vi "Measure.vi"(8 "Error In":errorcluster, 11 "Keithley 6482 In":refnum<visa-resource-name>) -> (0 "Error Out":errorcluster, 2 "Values":dbl[](array[numeric]), 3 "Keithley 6482 Out":refnum<visa-resource-name>)   [LabVIEW 2014, in "Keithley-6482-Visa.lvlib"]
uses:
  Keithley-6482-Visa.lvlib
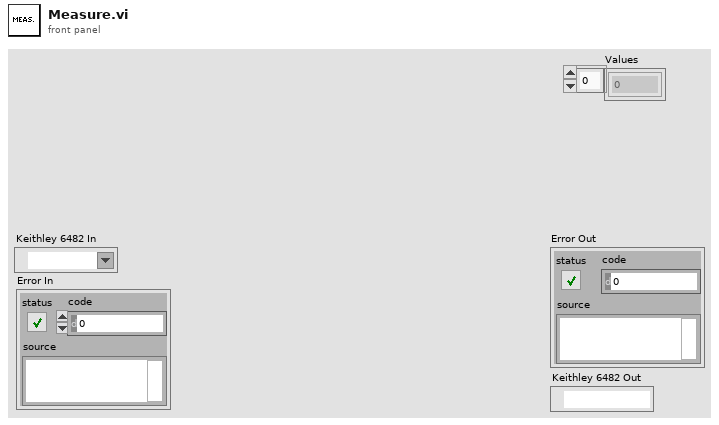
[diagram p1: front panel]
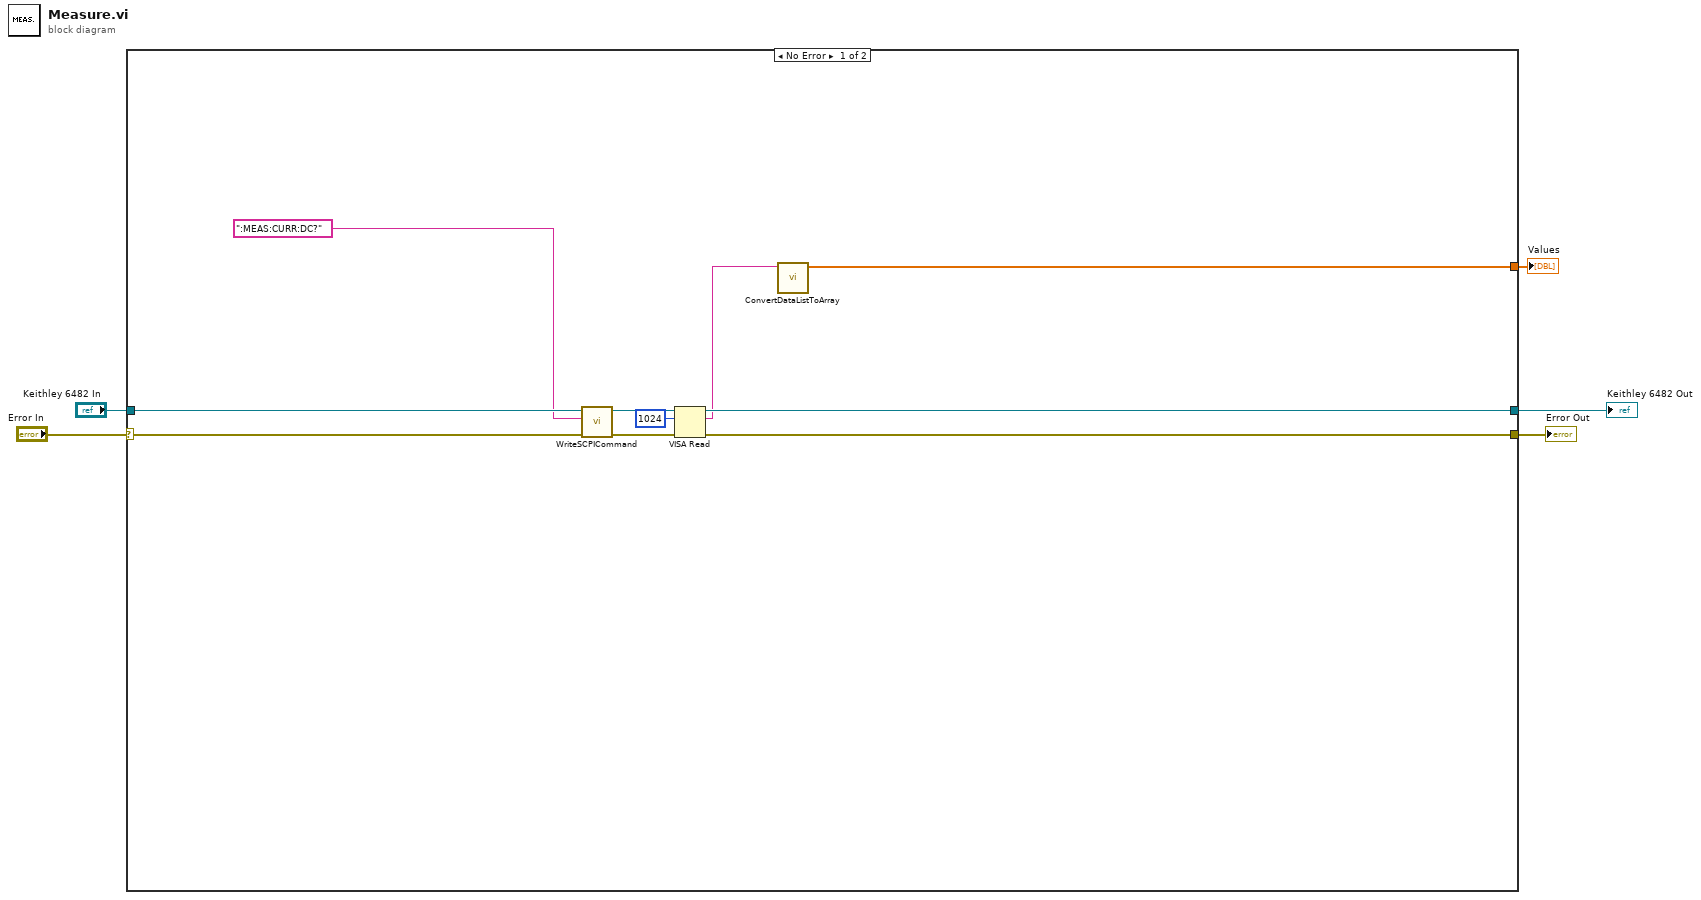
[diagram p0: block diagram]
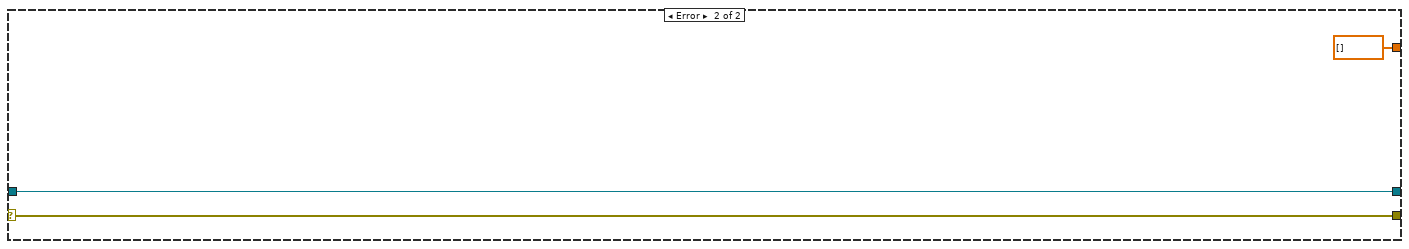
[diagram p2: hidden frame]
diagram:
  n1 = case shown="No Error" "Error In" {
    selector: "Error In" -> [w15 w17]
    tunnel: "Keithley 6482 In" -> [w14 w18]
    tunnel: [w10 w17] -> w3
    tunnel: [w9 w18] -> w2
    tunnel: [w6 dbl[] [] ("Values")] -> w1
    frame No Error {
      n2 = call "WriteSCPICommand.vi"("Error In"=w15, "SCPI Command"=":MEAS:CURR:DC?" ("string"), "Keithley 6482 In"=w14) -> ("Error Out"=w11:errorcluster, "Keithley 6482 Out"=w12:refnum<visa-resource-name>)  [unwired: 7 in]
      n3 = VISA Read(VISA resource name=w12, byte count=u32 1024, error in (no error)=w11) -> (VISA resource name out=w9:refnum<visa-resource-name>, read buffer=w7:string, error out=w10:errorcluster)  [unwired: 1 out]
      n4 = call "ConvertDataListToArray.vi"("Data List"=w7) -> ("Values"=w6:dbl[])  [unwired: 10 in]
    }
    frame Error {
    }
  }
  "Error Out" <- w3
  "Keithley 6482 Out" <- w2
  "Values" <- w1
